vi "ConvertTo_DBL.vi"(6 "Input Range (mV)":u32=10000, 7 "DC Offset (mV)":i32, 8 "Offset":i16, 9 "Resolution":i32=-32768, 10 "Interger Signal":i32[](array[numeric])) -> (2 "Data (V)":sgl[](array[numeric]) format="%.2f")   [LabVIEW 2013, in "Gage.lvlib"]
uses:
  <instrlib>/GageLv_uic/Gage.lvlib
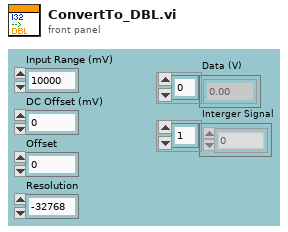
[diagram p1: front panel]
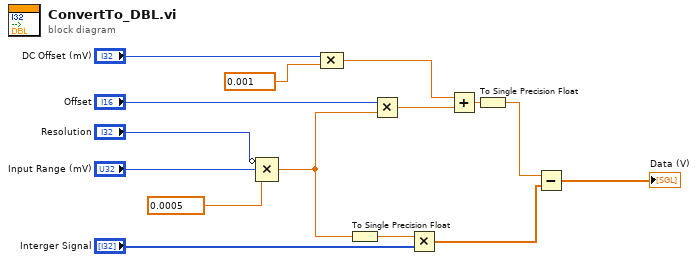
[diagram p0: block diagram]
diagram:
  n1 = Compound Arithmetic op=MULTIPLY(invert "Resolution", "Input Range (mV)", 0.0005) -> (w3:dbl)
  n2 = Compound Arithmetic op=MULTIPLY("DC Offset (mV)", 0.001) -> (w6:dbl)
  n3 = To Single Precision Float(number=w3) -> (single precision float=w2:sgl)
  n4 = Multiply(x="Offset", y=w3) -> (x*y=w7:dbl)
  n5 = Multiply(x=w2, y="Interger Signal") -> (x*y=w5:sgl[])
  n6 = Add(x=w6, y=w7) -> (x+y=w4:dbl)
  n7 = To Single Precision Float(number=w4) -> (single precision float=w1:sgl)
  n8 = Subtract(x=w1, y=w5) -> (x-y=→"Data (V)":sgl[])
